vi "IV(H)_DC_vector_magnet_fieldsweep_criticalcurrent_limited_BF_LD-400_K6221_K2182A_PK.vi"() -> ()   [LabVIEW 2016]
uses:
  <vilib>/Math Plots/2D Math Plots/2D Compass/2D Compass XCtrl/2D Compass.xctl
  <vilib>/Math Plots/2D Math Plots/2D Compass/2D Compass Datatype/Public/Plot Helper (Vector).vi
  LabView_Switching exp/SubVI/Keithley 622x LV 8.0/Keithley 622x.lvlib
  <vilib>/Math Plots/2D Math Plots/2D Compass/2D Compass Datatype/2D Compass Datatype.lvclass
  <vilib>/Analysis/NI_AALPro.lvlib
panel:
  out "2D Compass":refnum<class "2D Plot Datatype.lvclass">[](xcontrol)
  in  "Set Compliance voltage (V)":dbl=2.0 min=0.0 step=0.1 format="%_3f"
  in  "Step 3":dbl[](array[numeric])=[1e-06, 1e-06, 1e-06] min=-3000.0 max=3000.0 format="%.1e"
  in  "To 3":dbl[](array[numeric])=[0.00022, -0.00022, 0.0] min=-3000.0 max=3000.0 format="%.1e"
  in  "From 3":dbl[](array[numeric])=[0.0, 0.00022, -0.00022] min=-3000.0 max=3000.0 format="%.1e"
  in  "wait (ms)":u32=50
  in  "Nanovoltmeter 2182a VISA":refnum<visa-resource-name>="GPIB0::7::INSTR"
  in  "Current source K6221 VISA":refnum<visa-resource-name>="GPIB0::12::INSTR"
  in  "Number Averaging":i32=1
  in  "Tab Control":enum32{"Page 1", "Page 2"}(tab)
  out "V vs I":cluster{dbl, "Field Reading":dbl}[](graph)
  out "V vs time":cluster{dbl, "Field Reading":dbl}[](graph)
  out "Magnetic Field Vector Angle":dbl=-0.0007063202353624877 format="%#_13g"
  out "Magnetic Field Vector magnitude (T)":dbl=0.04899569500372294 format="%#_13g"
  in  "From 2":dbl[](array[numeric])=[45.0] min=-3000.0 max=3000.0 format="%#.5f"
  in  "To 2":dbl[](array[numeric])=[45.0] min=-3000.0 max=3000.0 format="%#.5g"
  in  "Step 2":dbl[](array[numeric])=[1.0] min=-3000.0 max=3000.0 format="%.3g"
  in  "Wait time after each sweep(min)":dbl=1.0 format="%#_13g"
  out "Z-axis Magnetic Field (T)":string="-0.000000604\r\n"
  in  "Y-axis Field ramp rate (T/min)":string="0.01"
  in  "Z-axis Field ramp rate (T/min)":string="0.01"
  out "Z-axis (90 deg)":dbl(slide)=-6.04e-07 scale=0.0..3.0
  out "Y-Axis (0deg)":dbl(slide)=0.048995695 scale=0.0..3.0
  out "Y-axis Magnetic Field (T)":string="0.048995695\r\n"
  in  "Magnet IP Address Z-axis":string="169.254.103.241"
  in  "Magnet IP Address Y-axis":string="169.254.50.121"
  out "Resistance (ohm)":dbl=-inf format="%#_13g"
  out "Time (s)":dbl=12035.086 format="%#_13g"
  in  "Magnetic field stabilization time (s)":dbl=2.0 format="%#_13g"
  in  "Step":dbl[](array[numeric])=[0.001] min=-3000.0 max=3000.0 format="%.4g"
  in  "To":dbl[](array[numeric])=[0.05] min=-3000.0 max=3000.0 format="%.4f"
  in  "From":dbl[](array[numeric])=[0.0] min=-3000.0 max=3000.0 format="%.4f"
  out "Iset (A)":dbl
  out "Vmeas (V)":dbl=-1.02396105e-06
  in  "Folder":path=path "D:/Banabir/sixth_round/20-10-2021"
  out "data":dbl[](array[numeric])=[0.04899569500372294, -0.0007063202353624877, 0.0, -1.02396105e-06, -inf, 12035.086]
  in  "File name":string="005_NTJJ01_250nmdevice_DC_IV_baseT_fieldsweep_I87_V56_1ave_nopreamp_45deg"
  out "File path":path=path "D:/Banabir/sixth_round/20-10-2021/004_NTJJ01_250nmdevice_DC_IV_baseT_fieldsweep_I87_V56_1ave_nopreamp.dat"
  # "Z-Axis: In-plane (90 deg)\nY-axis: Out-of-plane (0 deg)"
  # "[Must be less than 0.05]"
  # ".dat"
  # "It is important that there is enough time for the magnet to cool down after each sweep (Typically 15-20 min)"
  # "Configure Field Angle (deg)"
  # "Configure Field magnitude (T)"
  # "Configure current sweeps (A)"
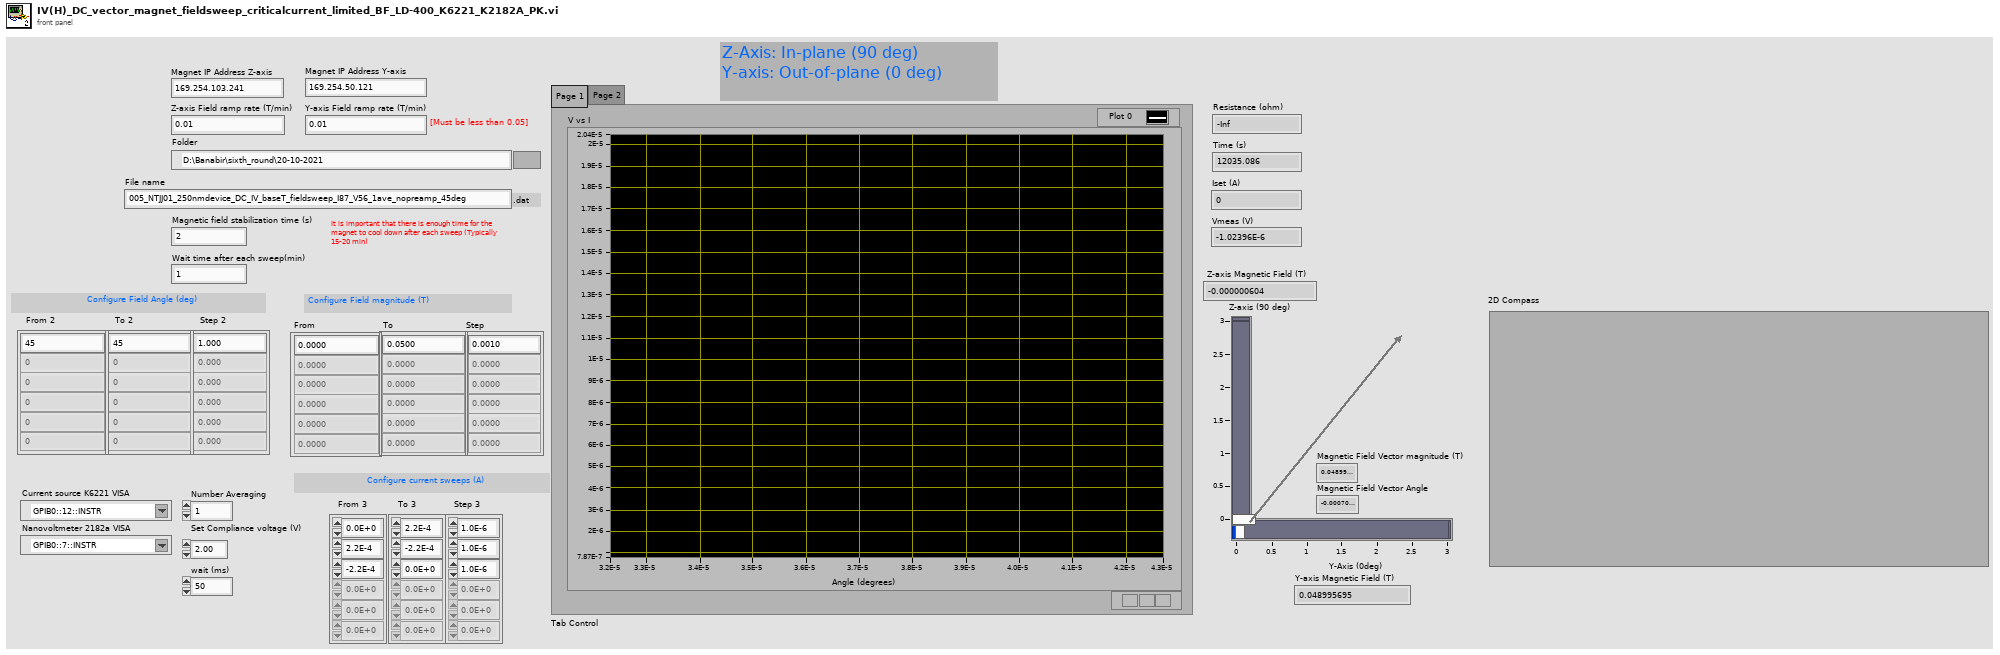
[diagram p1: front panel]
types:
  T1 = enum16{"open", "replace", "create", "open or create", "replace or create", "replace or create with confirmation"}
  T2 = typedef "Keithley 622x.lvlib/KE622x -- Current Level.ctl" = dbl
  T3 = cluster{"Average value":dbl, "Average value":dbl}
  T4 = cluster{"Average value":dbl, "Average value":dbl}[]
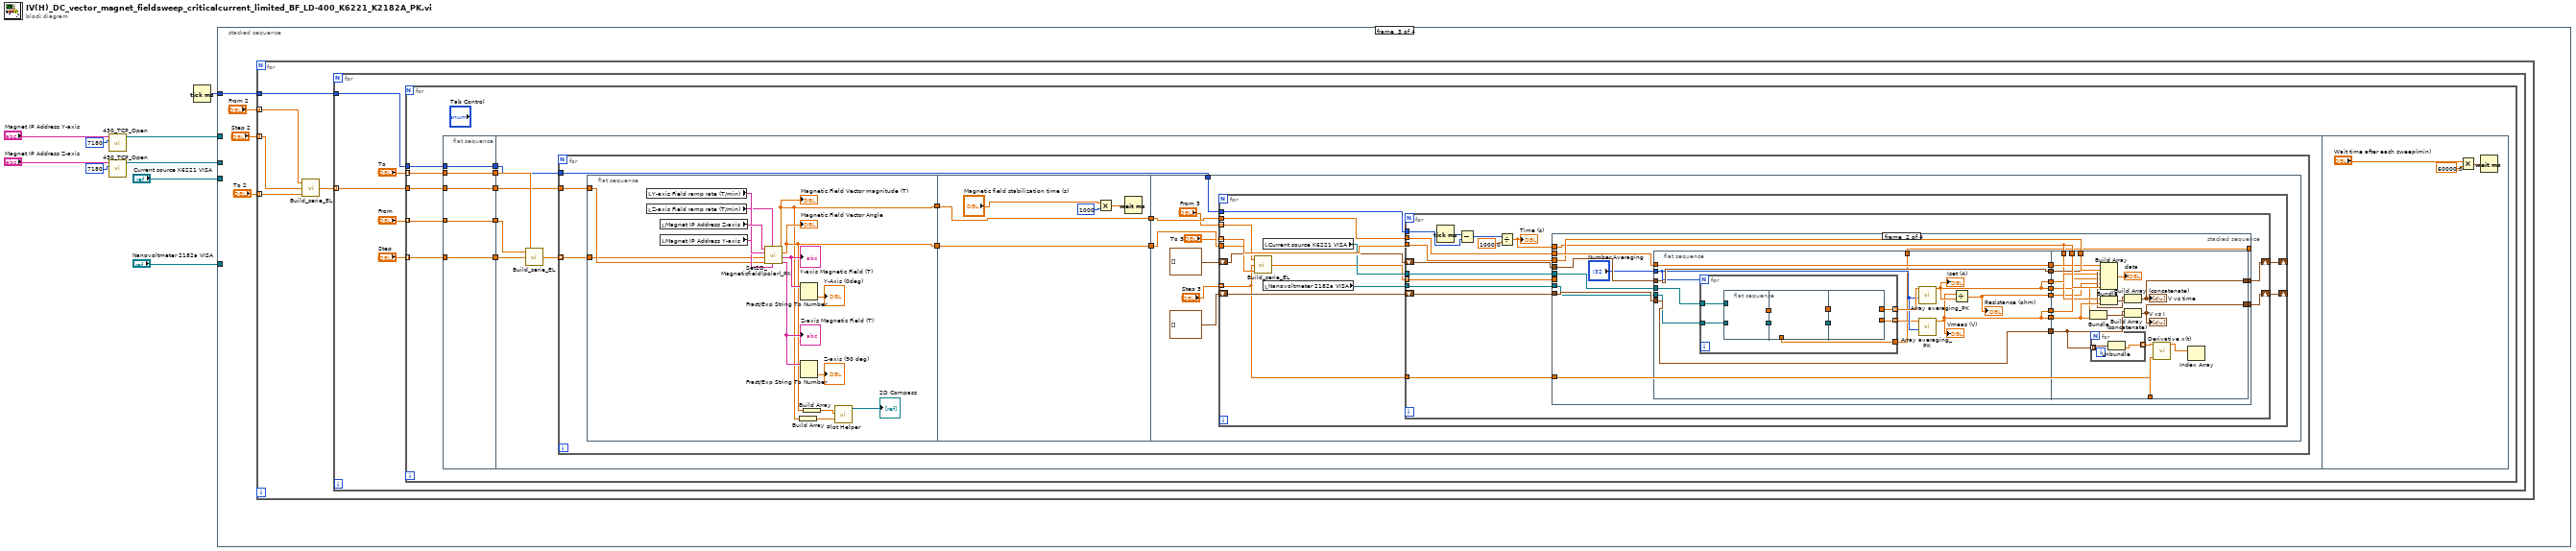
[diagram p0: block diagram]
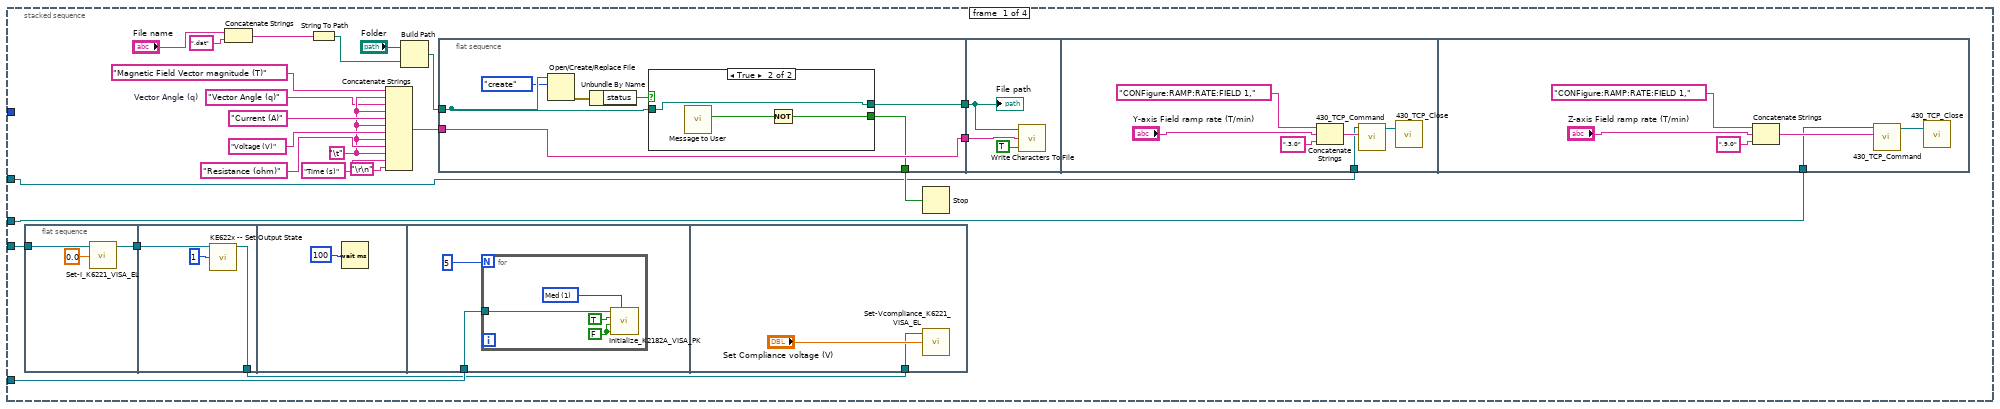
[diagram p2: hidden frame]
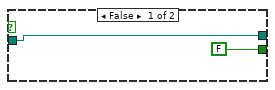
[diagram p3: hidden frame]
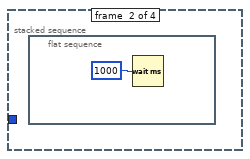
[diagram p4: hidden frame]
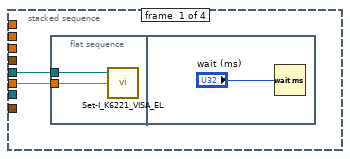
[diagram p5: hidden frame]
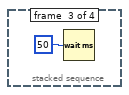
[diagram p6: hidden frame]
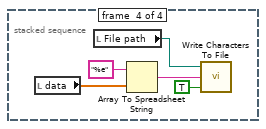
[diagram p7: hidden frame]
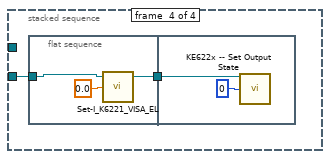
[diagram p8: hidden frame]
diagram:
  n1 = call "430_TCP_Open.vi"("IP Address"="Magnet IP Address Y-axis", "TCP Port"=7180) -> ("connection ID"=w8:refnum<k5>)  [unwired: 4 in, 2 out]
  n2 = call "430_TCP_Open.vi"("IP Address"="Magnet IP Address Z-axis", "TCP Port"=7180) -> ("connection ID"=w3:refnum<k5>)  [unwired: 4 in, 2 out]
  n3 = Tick Count (ms)() -> (millisecond timer value=w7:u32)
  n4 = stacked-sequence {
    tunnel: w8 -> [w19 _ _ _]
    tunnel: w7 -> [_ _ w80 _]
    tunnel: w3 -> [w16 _ _ _]
    tunnel: "Current source K6221 VISA" -> [w12 _ _ w260]
    tunnel: "Nanovoltmeter 2182a VISA" -> [w11 _ _ _]
    frame #0 {
      w14 = "Vector Angle (q)"  # Vector Angle (q)
      w15 = "\t"
      n5 = flat-sequence {
        tunnel: w12 -> [w36]
        tunnel: [w34] -> w13
        tunnel: w13 -> [w39]
        tunnel: [w37] -> w10
        tunnel: w11 -> [w41]
        tunnel: w10 -> [w47]
        frame #0 {
          n6 = call "Set-I_K6221_VISA_EL.vi"("Set I (A)"=0.0, "K6221 VISA"=w36) -> ("K6221 VISA out"=w34:refnum<visa-resource-name>)  [unwired: 2 in, 1 out]
        }
        frame #1 {
          n7 = call "KE622x -- Set Output State.vi"("Resource In"=w39, "Output State"=1) -> ("Resource Out (dupl)"=w37:refnum<visa-resource-name>)  [unwired: 12 in, 1 out]
        }
        frame #2 {
          n8 = Wait (ms)(milliseconds to wait=100) -> ()  [unwired: 1 out]
        }
        frame #3 {
          n9 = for {
            N: 5 ("Numeric") -> [_]
            tunnel: w41 -> [w43]
            w45 = u16 1 items=["Slow", "Med", "Fast"] ("Rate (NPLC)")
            w46 = FALSE ("Auto range?")
            n10 = call "Initialize_K2182A_VISA_PK.vi"("VISA address"=w43, "Auto range?"=TRUE, "Analog LPass\nFilter?"=w46, "DC\nFilter?"=w46, "Rate (NPLC)"=w45) -> ()  [unwired: 2 in]
          }
        }
        frame #4 {
          n11 = call "Set-Vcompliance_K6221_VISA_EL.vi"("Set Compliance voltage (V)"="Set Compliance voltage (V)", "K6221 VISA"=w47) -> ()  [unwired: 2 in, 2 out]
        }
      }
      n12 = Concatenate Strings("File name", ".dat" ("string")) -> (w29:string)
      n13 = String To Path(string=w29) -> (path=w21:path)
      n14 = Concatenate Strings("Magnetic Field Vector magnitude (T)", w15, w14, w15, "Current (A)" ("string"), w15, "Voltage (V)" ("string"), w15, "Resistance (ohm)" ("string"), w15, "Time (s)", "\r\n") -> (w30:string)
      n15 = Build Path(base path="Folder", name or relative path=w21) -> (appended path=w20:path)
      n16 = flat-sequence {
        tunnel: w20 -> [w52]
        tunnel: w30 -> [w55]
        tunnel: [w55] -> w33
        tunnel: [w54] -> w27
        tunnel: [w53] -> w32
        tunnel: w33 -> [w62]
        tunnel: w32 -> [w61]
        tunnel: w19 -> [w65]
        tunnel: w16 -> [w70]
        frame #0 {
          n17 = Open/Create/Replace File(file path (use dialog)=w52, operation (0:open)=T1."create") -> (error out=w51:errorcluster)  [unwired: 4 in, 2 out]
          n18 = Unbundle By Name(w51) -> ("status"=w49:bool)
          n19 = case shown="True" w49 {
            tunnel: [FALSE ("Yes") w59] -> w54
            tunnel: [w56 w58] -> w53
            tunnel: w52 -> [w56 w58]
            frame False {
            }
            frame True {
              n20 = call "Message to User"() -> ("Yes"=w60:bool)  [unwired: 10 in, 1 out]
              n21 = Not(x=w60) -> (.not. x?=w59:bool)
            }
          }
        }
        frame #1 {
          n22 = call <vilib>:"Write Characters To File.vi"("append to file? (new file:F)"=TRUE, "character string"=w62, "file path (dialog if empty)"=w61) -> ()  [unwired: 2 in, 1 out]
          "File path" <- w61
        }
        frame #2 {
          n23 = Concatenate Strings("CONFigure:RAMP:RATE:FIELD 1," ("String"), "Y-axis Field ramp rate (T/min)", ",3.0") -> (w66:string)
          n24 = call "430_TCP_Command.vi"("Command"=w66, "connection ID"=w65) -> ("connection ID out"=w69:refnum<k5>)  [unwired: 2 in, 2 out]
          n25 = call "430_TCP_Close.vi"("connection ID"=w69) -> ()  [unwired: 1 in, 2 out]
        }
        frame #3 {
          n26 = Concatenate Strings("CONFigure:RAMP:RATE:FIELD 1," ("String"), "Z-axis Field ramp rate (T/min)", ",9.0") -> (w72:string)
          n27 = call "430_TCP_Command.vi"("Command"=w72, "connection ID"=w70) -> ("connection ID out"=w75:refnum<k5>)  [unwired: 2 in, 2 out]
          n28 = call "430_TCP_Close.vi"("connection ID"=w75) -> ()  [unwired: 1 in, 2 out]
        }
      }
      n29 = Stop(stop? (T)=w27) -> ()
    }
    frame #1 {
      n30 = flat-sequence {
        frame #0 {
          n31 = Wait (ms)(milliseconds to wait=u32 1000) -> ()  [unwired: 1 out]
        }
      }
    }
    frame #2 {
      n32 = for {
        tunnel: w80 -> [w85]
        tunnel: "From 2" -> [w84] mode=indexing
        tunnel: "To 2" -> [w83] mode=indexing
        tunnel: "Step 2" -> [w82] mode=indexing
        n33 = call "Build_serie_EL.vi"("end value"=w83, "increment"=w82, "start value"=w84) -> ("output array"=w81:dbl[])
        n34 = for {
          tunnel: w85 -> [w87]
          tunnel: w81 -> [w86] mode=indexing
          n35 = for {
            tunnel: "From" -> [w100] mode=indexing
            tunnel: "To" -> [w98] mode=indexing
            tunnel: "Step" -> [w99] mode=indexing
            tunnel: w87 -> [w97]
            tunnel: w86 -> [w92]
            n36 = flat-sequence {
              tunnel: w97 -> [w102]
              tunnel: w98 -> [w103]
              tunnel: w99 -> [w104]
              tunnel: w100 -> [w105]
              tunnel: [w105] -> w96
              tunnel: [w104] -> w95
              tunnel: [w103] -> w94
              tunnel: [w102] -> w93
              tunnel: w92 -> [w101]
              tunnel: [w101] -> w91
              tunnel: w96 -> [w111]
              tunnel: w95 -> [w110]
              tunnel: w94 -> [w109]
              tunnel: w93 -> [w107]
              tunnel: w91 -> [w106]
              frame #0 {
              }
              frame #1 {
                n37 = call "Build_serie_EL.vi"("end value"=w109, "increment"=w110, "start value"=w111) -> ("output array"=w108:dbl[])
                n38 = for {
                  tunnel: w108 -> [w118] mode=indexing
                  tunnel: w107 -> [w117]
                  tunnel: w106 -> [w116]
                  n39 = flat-sequence {
                    tunnel: [w119] -> w115
                    tunnel: [w120] -> w112
                    tunnel: w116 -> [w125]
                    tunnel: w118 -> [w124]
                    tunnel: w115 -> [w135]
                    tunnel: [w135] -> w114
                    tunnel: [w134] -> w113
                    tunnel: w112 -> [w134]
                    tunnel: w113 -> [w144]
                    tunnel: w114 -> [w145]
                    tunnel: w117 -> [w146]
                    frame #0 {
                      n40 = local read "Y-axis Field ramp rate (T/min)"() -> (w131:string)
                      n41 = local read "Z-axis Field ramp rate (T/min)"() -> (w130:string)
                      n42 = local read "Magnet IP Address Z-axis"() -> (w133:string)
                      n43 = local read "Magnet IP Address Y-axis"() -> (w132:string)
                      n44 = call "Set2D_Magneticfield(polar)_PK.vi"("Y-axis Ramp Rate (T/min)"=w131, "Z-axis Ramp Rate (T/min)"=w130, "Set target vector angle (degrees)"=w125, "Set target vector magnitude (T)"=w124, "Y-Axis Magnet IP Address"=w132, "Z-Axis Magnet IP Address"=w133) -> ("Z-axis Magnetic Field (T)"=w127:string, "Y-axis Magnetic Field (T)"=w129:string, "q - Vector angle"=w120:dbl, "R - Vector field magnitude (T)"=w119:dbl)  [unwired: 2 in]
                      "Z-axis Magnetic Field (T)" <- w127
                      "Y-axis Magnetic Field (T)" <- w129
                      "Magnetic Field Vector magnitude (T)" <- w119
                      "Magnetic Field Vector Angle" <- w120
                      n45 = Build Array(w119) -> (w122:dbl[])
                      n46 = Fract/Exp String To Number(string=w129) -> (number=→"Y-Axis (0deg)":dbl)  [unwired: 3 in, 1 out]
                      n47 = Fract/Exp String To Number(string=w127) -> (number=→"Z-axis (90 deg)":dbl)  [unwired: 3 in, 1 out]
                      n48 = Build Array(w120) -> (w121:dbl[])
                      n49 = call-poly <vilib>:"Plot Helper.vi"("radius vector"=w122, "theta vector"=w121) -> ("2D Plot Class Obj Array out"=→"2D Compass":refnum<class "2D Plot Datatype.lvclass">[])  [unwired: 2 in, 7 out]
                    }
                    frame #1 {
                      n50 = Multiply(x="Magnetic field stabilization time (s)", y=1000) -> (x*y=w137:dbl)
                      n51 = Wait (ms)(milliseconds to wait=w137) -> ()  [unwired: 1 out]
                    }
                    frame #2 {
                      n52 = for {
                        tunnel: w146 -> [w159]
                        tunnel: w145 -> [w157]
                        tunnel: w144 -> [w156]
                        tunnel: "From 3" -> [w151] mode=indexing
                        tunnel: "Step 3" -> [w147] mode=indexing
                        tunnel: "To 3" -> [w150] mode=indexing
                        shift-right: [w149] -> _
                        shift-left: cluster{dbl, "Field Reading":dbl}[] [] -> [w155]
                        shift-right: [w148] -> _
                        shift-left: cluster{dbl, "Field Reading":dbl}[] [] -> [w158]
                        n53 = call "Build_serie_EL.vi"("end value"=w150, "increment"=w147, "start value"=w151) -> ("output array"=w152:dbl[])
                        n54 = local read "Current source K6221 VISA"() -> (w154:refnum<visa-resource-name>)
                        n55 = local read "Nanovoltmeter 2182a VISA"() -> (w153:refnum<visa-resource-name>)
                        n56 = for {
                          tunnel: w159 -> [w174]
                          tunnel: w157 -> [w168]
                          tunnel: w156 -> [w167]
                          tunnel: w152 -> [w165] mode=indexing
                          shift-right: [w161] -> w148
                          shift-left: w158 -> [w173]
                          shift-right: [w162] -> w149
                          shift-left: w155 -> [w166]
                          tunnel: w154 -> [w164]
                          tunnel: w153 -> [w163]
                          tunnel: w147 -> [w160]
                          n57 = Tick Count (ms)() -> (millisecond timer value=w170:u32)
                          n58 = Subtract(x=w170, y=w174) -> (x-y=w172:u32)
                          n59 = Divide(x=w172, y=1000.0) -> (x/y=w169:dbl)
                          "Time (s)" <- w169
                          n60 = stacked-sequence {
                            tunnel: w173 -> [_ w198 _ _]
                            tunnel: [_ w199 _ _] -> w161
                            tunnel: w169 -> [_ w186 _ _]
                            tunnel: w168 -> [_ w193 _ _]
                            tunnel: w167 -> [_ w192 _ _]
                            tunnel: [_ w191 _ _] -> w162
                            tunnel: w166 -> [_ w189 _ _]
                            tunnel: w165 -> [w176 _ _ _]
                            tunnel: [_ w183 _ _] -> _
                            tunnel: w164 -> [w175 w182 _ _]
                            tunnel: w163 -> [_ w181 _ _]
                            tunnel: w160 -> [_ w180 _ _]
                            frame #0 {
                              n61 = flat-sequence {
                                tunnel: w176 -> [w178]
                                tunnel: w175 -> [w177]
                                frame #0 {
                                n62 = call "Set-I_K6221_VISA_EL.vi"("Set I (A)"=w178, "K6221 VISA"=w177) -> ()  [unwired: 2 in, 2 out]
                                }
                                frame #1 {
                                n63 = Wait (ms)(milliseconds to wait="wait (ms)") -> ()  [unwired: 1 out]
                                }
                              }
                            }
                            frame #1 {
                              n64 = flat-sequence {
                                tunnel: [w205] -> w197
                                tunnel: [w211] -> w196
                                tunnel: [w207] -> w195
                                tunnel: [w210] -> w194
                                tunnel: [w209] -> w190
                                tunnel: "Number Averaging" -> [w204]
                                tunnel: w189 -> [w209]
                                tunnel: w198 -> [w211]
                                tunnel: w193 -> [w210]
                                tunnel: [w205] -> w187
                                tunnel: [w207] -> w185
                                tunnel: [w208] -> w184
                                tunnel: [w202] -> w183
                                tunnel: w182 -> [w201]
                                tunnel: w181 -> [w200]
                                tunnel: w197 -> [w238]
                                tunnel: [w247] -> w199
                                tunnel: w196 -> [w233]
                                tunnel: w195 -> [w237]
                                tunnel: w194 -> [w242]
                                tunnel: w186 -> [w245]
                                tunnel: w192 -> [w244]
                                tunnel: [w240] -> w191
                                tunnel: w190 -> [w239]
                                tunnel: w187 -> [w241]
                                tunnel: w186 -> [w236]
                                tunnel: w185 -> [w235]
                                tunnel: w184 -> [w234]
                                tunnel: w180 -> [w231]
                                frame #0 {
                                n65 = for {
                                N: w204 -> [_]
                                tunnel: [w213] -> w203 mode=indexing
                                tunnel: [w212] -> w206 mode=indexing
                                tunnel: w201 -> [w219]
                                tunnel: [w218] -> w202
                                tunnel: w200 -> [w220]
                                n66 = flat-sequence {
                                tunnel: w219 -> [w221]
                                tunnel: w220 -> [w223]
                                tunnel: [w223] -> w217
                                tunnel: [w222] -> w216
                                tunnel: [w225] -> w218
                                tunnel: w217 -> [w226]
                                tunnel: w216 -> [w225]
                                tunnel: [w226] -> w215
                                tunnel: [w225] -> w214
                                tunnel: [w229] -> w212
                                tunnel: w215 -> [w228]
                                tunnel: w214 -> [w229]
                                tunnel: [w227] -> w213
                                frame #0 {
                                n67 = call "KE622x -- Get Current Level.vi"("Resource In"=w221) -> ("Current Level (A)"=w222:T2)  [unwired: 12 in, 2 out]
                                }
                                frame #1 {
                                n68 = Wait (ms)(milliseconds to wait=50) -> ()  [unwired: 1 out]
                                }
                                frame #2 {
                                n69 = call "Get-V_K2182A_VISA_EL.vi"("VISA K2182A"=w228) -> ("V (V)"=w227:dbl)  [unwired: 2 in, 2 out]
                                }
                                }
                                }
                                n70 = call "Array averaging_PK.vi"("Number averaging"=w204, "numeric array"=w206) -> ("Average value"=w207:dbl)  [unwired: 9 in]
                                "Iset (A)" <- w207
                                n71 = call "Array averaging_PK.vi"("Number averaging"=w204, "numeric array"=w203) -> ("Average value"=w205:dbl)  [unwired: 9 in]
                                "Vmeas (V)" <- w205
                                n72 = Divide(x=w205, y=w207) -> (x/y=w208:dbl)
                                "Resistance (ohm)" <- w208
                                }
                                frame #1 {
                                n73 = Bundle("Average value"=w235, "Average value"=w241) -> (w246:T3)  [unwired: 1 in]
                                n74 = for {
                                tunnel: w233 -> [w250] mode=indexing
                                tunnel: [w249] -> w232 mode=indexing
                                n75 = Unbundle(w250) -> ("Field Reading"=w249:dbl)  [unwired: 1 out]
                                }
                                n76 = Build Array(w242, w244, w237, w238, w234, w245) -> (→"data":dbl[])
                                n77 = Bundle(w236, "Average value"=w241) -> (w243:cluster{dbl, "Average value":dbl})  [unwired: 1 in]
                                n78 = Build Array (concatenate)(w239, w243) -> (w240:cluster{dbl, "Average value":dbl}[])
                                "V vs time" <- w240
                                n79 = Build Array (concatenate)(w233, w246) -> (w247:T4)
                                "V vs I" <- w247
                                n80 = call <vilib>:"Derivative x(t).vi"("dt"=w231, "X"=w232) -> ("dX/dt"=w230:dbl[])  [unwired: 8 in, 1 out]
                                n81 = Index Array(array=w230) -> ()  [unwired: 1 in, 1 out]
                                }
                              }
                            }
                            frame #2 {
                              n82 = Wait (ms)(milliseconds to wait=u32 50) -> ()  [unwired: 1 out]
                            }
                            frame #3 {
                              n83 = local read "data"() -> (w252:dbl[])
                              n84 = local read "File path"() -> (w254:path)
                              n85 = Array To Spreadsheet String(array=w252, 3:"%e" ("format string")) -> (spreadsheet string=w255:string)  [unwired: 1 in]
                              n86 = call <vilib>:"Write Characters To File.vi"("append to file? (new file:F)"=TRUE, "character string"=w255, "file path (dialog if empty)"=w254) -> ()  [unwired: 2 in, 1 out]
                            }
                          }
                        }
                      }
                    }
                  }
                }
              }
              frame #2 {
                n87 = Multiply(x="Wait time after each sweep(min)", y=60000.0) -> (x*y=w259:dbl)
                n88 = Wait (ms)(milliseconds to wait=w259) -> ()  [unwired: 1 out]
              }
            }
          }
        }
      }
    }
    frame #3 {
      n89 = flat-sequence {
        tunnel: w260 -> [w264]
        tunnel: [w262] -> w261
        tunnel: w261 -> [w266]
        frame #0 {
          n90 = call "Set-I_K6221_VISA_EL.vi"("Set I (A)"=0.0, "K6221 VISA"=w264) -> ("K6221 VISA out"=w262:refnum<visa-resource-name>)  [unwired: 2 in, 1 out]
        }
        frame #1 {
          n91 = call "KE622x -- Set Output State.vi"("Resource In"=w266, "Output State"=0) -> ()  [unwired: 12 in, 2 out]
        }
      }
    }
  }
